vi "40 Config File Path (x64-2018).vi"() -> (0 "Configuration File Path":path)   [LabVIEW 2017]
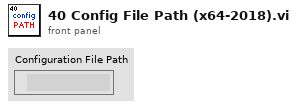
[diagram p1: front panel]
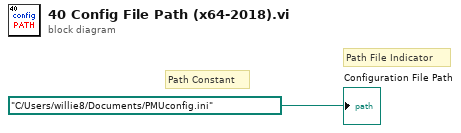
[diagram p0: block diagram]
diagram:
  # "Path File Indicator"
  # "Path Constant"
  "Configuration File Path" <- path "C:/Users/willie8/Documents/PMUconfig.ini"
